vi "Arc Length of Bezier Spline 2.vi"(10 "ctrl pts":cluster{"x":sgl, "y":sgl}[][](array[cluster]), 11 "position":sgl[][](array[numeric])) -> (2 "l total":dbl, 3 "l":dbl[](array[numeric]))   [LabVIEW 2019]
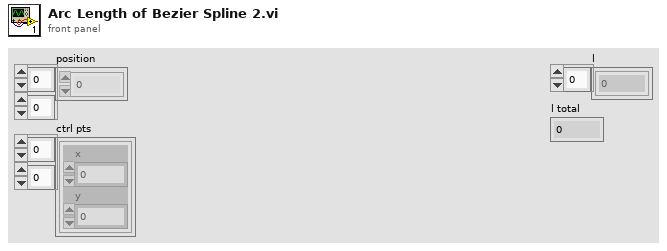
[diagram p1: front panel]
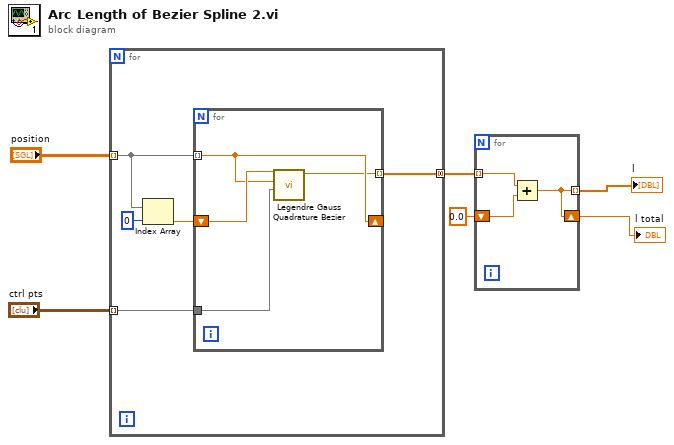
[diagram p0: block diagram]
diagram:
  n1 = for {
    tunnel: "position" -> [w10] mode=indexing
    tunnel: "ctrl pts" -> [w8] mode=indexing
    tunnel: [w7] -> w4 mode=concatenating
    n2 = Index Array(array=w10, index=0) -> (element=w11:sgl)
    n3 = for {
      tunnel: w10 -> [w14] mode=indexing
      shift-right: [w14] -> _
      shift-left: w11 -> [w15]
      tunnel: w8 -> [w13]
      tunnel: [w12] -> w7 mode=indexing
      n4 = call "Legendre Gauss Quadrature Bezier.vi"("ctrl points"=w13, "t1"=w14, "t0"=w15) -> ("l"=w12:dbl)  [unwired: 8 in]
    }
  }
  n5 = for {
    tunnel: w4 -> [w18] mode=indexing
    shift-right: [w16] -> w1
    shift-left: 0.0 ("l total") -> [w17]
    tunnel: [w16] -> w2 mode=indexing
    n6 = Add(x=w18, y=w17) -> (x+y=w16:dbl)
  }
  "l" <- w2
  "l total" <- w1
